vi "Zad1.vi"() -> ()   [LabVIEW 2015]
uses:
  <vilib>/DAQmx/write.llb/DAQmx Write (Analog 1D DBL 1Chan NSamp).vi
  <vilib>/DAQmx/read.llb/DAQmx Read (Analog 1D DBL 1Chan NSamp).vi
  <vilib>/DAQmx/create/channels.llb/DAQmx Create Channel (AO-Voltage-Basic).vi
  <vilib>/DAQmx/configure/timing.llb/DAQmx Timing (Sample Clock).vi
  <vilib>/DAQmx/miscellaneous.llb/DAQmx Fill In Error Info.vi
  <vilib>/DAQmx/create/channels.llb/DAQmx Create Channel (AI-Voltage-Basic).vi
  <vilib>/ptbypt/NI_PtbyPt.lvlib
panel:
  out "error out":errorcluster
  in  "physical channels":tag
  in  "OK Button":bool
  out "Waveform Chart":dbl[](graph)
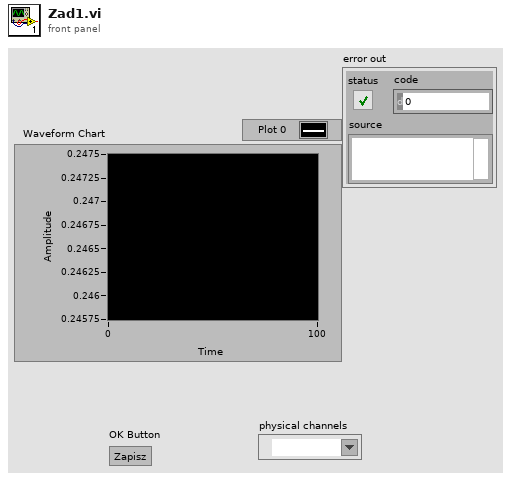
[diagram p1: front panel]
types:
  T1 = enum16{"open", "replace", "create", "open or create", "replace or create", "replace or create with confirmation"}
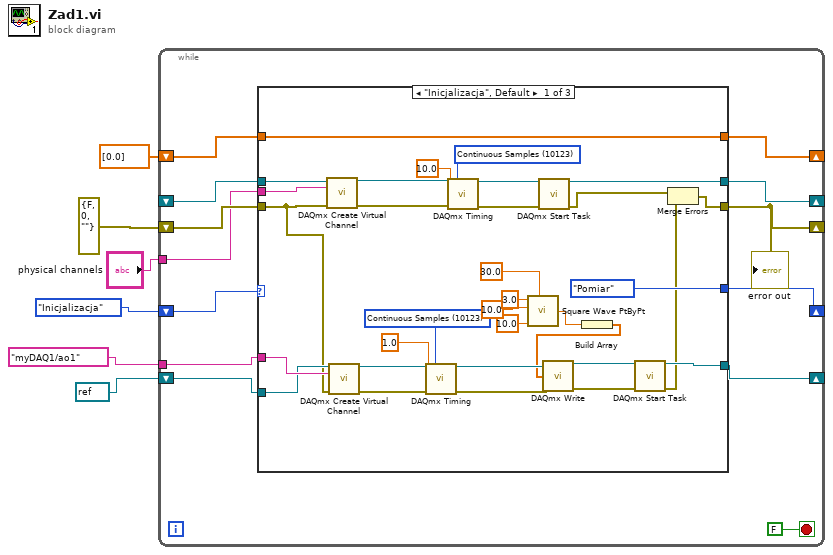
[diagram p0: block diagram]
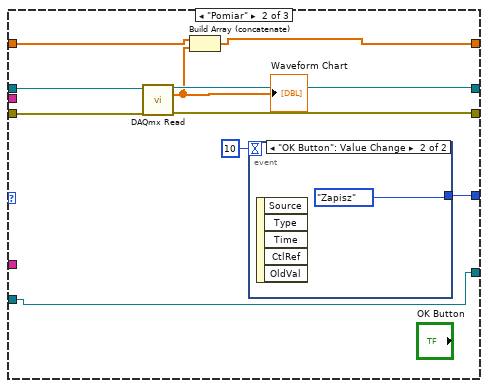
[diagram p2: hidden frame]
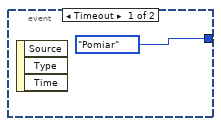
[diagram p3: hidden frame]
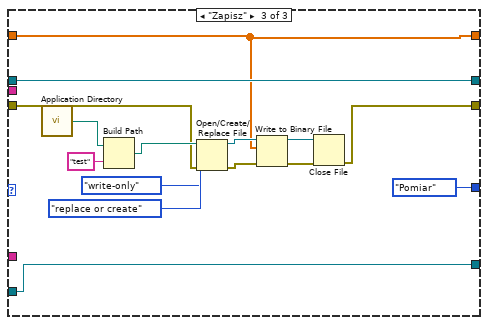
[diagram p4: hidden frame]
diagram:
  n1 = while {
    shift-right: [w16] -> _
    shift-left: _ -> [w15]
    shift-right: [w14] -> _
    shift-left: errorcluster {"status"=FALSE, "code"=0, "source"=""} ("error constant") -> [w17]
    shift-right: [w13] -> _
    shift-left: enum16{"Zapisz", "Pomiar", "Inicjalizacja"}."Inicjalizacja" -> [w18]
    shift-right: [w12] -> _
    shift-left: dbl[] [0.0] ("data") -> [w11]
    tunnel: "physical channels" -> [w10]
    shift-right: [w8] -> _
    shift-left: refnum<k21> refnum ("task in") -> [w9]
    tunnel: tag "myDAQ1/ao1" ("physical channels") -> [w7]
    stop <- FALSE stop-if-true
    n2 = case shown="\"Inicjalizacja\", Default" w18 {
      tunnel: w17 -> [w26 w60 w73]
      tunnel: [w47 w59 w77] -> w16
      tunnel: w15 -> [w41 w61 w77]
      tunnel: [w20 w58 w68] -> w14
      tunnel: [enum16{"Zapisz", "Pomiar", "Inicjalizacja"}."Pomiar" w56 enum16{"Zapisz", "Pomiar", "Inicjalizacja"}."Pomiar"] -> w13
      tunnel: [w42 w53 w67] -> w12
      tunnel: w11 -> [w42 w55 w67]
      tunnel: w10 -> [w43 _ _]
      tunnel: w7 -> [w40 _ _]
      tunnel: w9 -> [w39 w52 w64]
      tunnel: [w35 w52 w64] -> w8
      frame "Inicjalizacja", Default {
        w36 = 10123 items=["Finite Samples"=10178, "Continuous Samples"=10123, "Hardware Timed Single Point"=12522] ("sample mode")
        w46 = 10123 items=["Finite Samples"=10178, "Continuous Samples"=10123, "Hardware Timed Single Point"=12522] ("sample mode")
        n3 = call-poly <vilib>:"DAQmx Create Virtual Channel.vi"("task in"=w41, "physical channels"=w43, "error in"=w26) -> ("task out"=w51:refnum<k21>, "error out"=w49:errorcluster)  [unwired: 11 in]
        n4 = call-poly <vilib>:"DAQmx Create Virtual Channel.vi"("task in"=w39, "physical channels"=w40, "error in"=w26) -> ("task out"=w38:refnum<k21>, "error out"=w25:errorcluster)  [unwired: 11 in]
        n5 = call-poly <vilib>:"DAQmx Timing.vi"("task/channels in"=w38, "sample mode"=w36, "rate"=1.0, "error in"=w25) -> ("task out"=w34:refnum<k21>, "error out"=w24:errorcluster)  [unwired: 10 in]
        n6 = call-poly <vilib>:"DAQmx Timing.vi"("task/channels in"=w51, "sample mode"=w46, "rate"=10.0, "error in"=w49) -> ("task out"=w48:refnum<k21>, "error out"=w45:errorcluster)  [unwired: 10 in]
        n7 = call <vilib>:"Square Wave PtByPt.vi"("amplitude"=3.0, "frequency"=10.0, "time"=10.0, "duty cycle (%)"=30.0) -> ("square wave"=w28:dbl)  [unwired: 1 in]
        n8 = call <vilib>:"DAQmx Start Task.vi"("task/channels in"=w48, "error in"=w45) -> ("task out"=w47:refnum<k21>, "error out"=w22:errorcluster)  [unwired: 12 in]
        n9 = Build Array(w28) -> (w27:dbl[])
        n10 = call-poly <vilib>:"DAQmx Write.vi"("task/channels in"=w34, "data"=w27, "error in"=w24) -> ("task out"=w33:refnum<k21>, "error out"=w23:errorcluster)  [unwired: 10 in, 1 out]
        n11 = call <vilib>:"DAQmx Start Task.vi"("task/channels in"=w33, "error in"=w23) -> ("task out"=w35:refnum<k21>, "error out"=w21:errorcluster)  [unwired: 12 in]
        n12 = Merge Errors(w22, w21) -> (w20:errorcluster)
      }
      frame "Pomiar" {
        n13 = call-poly <vilib>:"DAQmx Read.vi"("task/channels in"=w61, "error in"=w60) -> ("task out"=w59:refnum<k21>, "data"=w54:dbl[], "error out"=w58:errorcluster)  [unwired: 11 in]
        "Waveform Chart" <- w54
        n14 = Build Array (concatenate)(w55, w54) -> (w53:dbl[])
        n15 = event shown="[1] \"OK Button\": Value Change" {
          selector: _ -> [_ _]
          dyn-events: _ -> [_ _]
          timeout: 10 -> [_ _]
          tunnel: [enum16{"Zapisz", "Pomiar", "Inicjalizacja"}."Pomiar" enum16{"Zapisz", "Pomiar", "Inicjalizacja"}."Zapisz"] -> w56
          event Timeout {
            n16 = event-data() -> ()  [unwired: 1 in, 3 out]
          }
          event "OK Button": Value Change {
            n17 = event-data() -> ()  [unwired: 1 in, 5 out]
          }
        }
      }
      frame "Zapisz" {
        n18 = call <vilib>:"Application Directory.vi"() -> ("Application Directory"=w76:path)
        n19 = Build Path(base path=w76, name or relative path="test") -> (appended path=w74:path)
        n20 = Open/Create/Replace File(file path (use dialog)=w74, error in=w73, operation (0:open)=T1."replace or create", access (0:read/write)=enum16{"read/write", "read-only", "write-only"}."write-only") -> (refnum out=w72:refnum<file>, error out=w71:errorcluster)  [unwired: 2 in, 1 out]
        n21 = Write to Binary File(file (use dialog)=w72, data=w67, error in=w71) -> (refnum out=w69:refnum<file>, error out=w70:errorcluster)  [unwired: 3 in, 1 out]
        n22 = Close File(refnum=w69, error in=w70) -> (error out=w68:errorcluster)  [unwired: 1 out]
      }
    }
    "error out" <- w14
  }
